vi "Group Reference Toggle.vi"(0 "Samples per Channel":i32, 1 "Show Reference":bool, 5 "Show Signal 1":bool, 7 "Show Signal 2":bool, 9 "Upper Voltage Threshold Reference":dbl, 11 "Upper Voltage Threshold Signal 1":dbl, 12 "Lower Voltage Threshold Reference":dbl, 13 "Upper Voltage Threshold Signal 2":dbl, 14 "Lower Voltage Threshold Signal 1":dbl, 15 "Lower Voltage Threshold Signal 2":dbl) -> (4 "Reference Signal 0":dbl[][](array[numeric]), 6 "Ref Signal 1":dbl[][](array[numeric]), 8 "Ref Signal 2":dbl[][](array[numeric]), 10 "Array":dbl[][](array[numeric]))   [LabVIEW 2009]
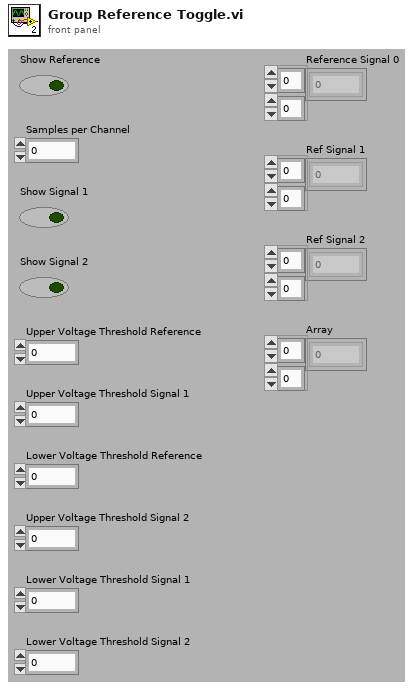
[diagram p1: front panel]
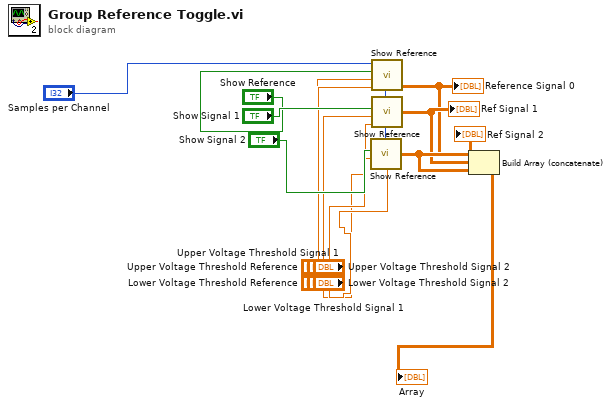
[diagram p0: block diagram]
diagram:
  n1 = call "Show Reference.vi"("Lower Voltage Threshold Reference"="Lower Voltage Threshold Signal 2", "Upper Voltage Threshold Reference"="Upper Voltage Threshold Signal 2", "Show Channel"="Show Signal 2", "Samples per Channel"="Samples per Channel") -> ("Reference Levels"=w13:dbl[][])
  "Ref Signal 2" <- w13
  n2 = call "Show Reference.vi"("Lower Voltage Threshold Reference"="Lower Voltage Threshold Reference", "Upper Voltage Threshold Reference"="Upper Voltage Threshold Reference", "Show Channel"="Show Reference", "Samples per Channel"="Samples per Channel") -> ("Reference Levels"=w11:dbl[][])
  "Reference Signal 0" <- w11
  n3 = call "Show Reference.vi"("Lower Voltage Threshold Reference"="Lower Voltage Threshold Signal 1", "Upper Voltage Threshold Reference"="Upper Voltage Threshold Signal 1", "Show Channel"="Show Signal 1", "Samples per Channel"="Samples per Channel") -> ("Reference Levels"=w12:dbl[][])
  "Ref Signal 1" <- w12
  n4 = Build Array (concatenate)(w11, w12, w13) -> (→"Array":dbl[][])
